vi "弹窗-手动静音.vi"(6 "引用-报警方式值改变？":refnum<vi>, 8 "引用-报警状态":refnum<vi>, 9 "引用-暂停发送":refnum<vi>, 10 "引用-报警方式":refnum<vi>, 11 "引用-实时数据列表":refnum<vi>) -> ()   [LabVIEW 2017]
panel:
  in  "列表框":i32(listbox)
  in  "事件-选中行":refnum<user-event>
  in  "选中行":i32[](array[numeric])
  out "项数":i32
  out "信号-刷新列表":bool=TRUE
  in  "上翻":bool
  in  "全部静音":bool
  in  "下翻":bool
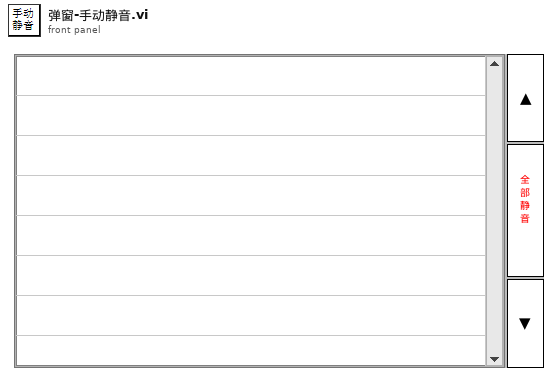
[diagram p1: front panel]
types:
  T1 = cluster{"报警方式":enum16{"常报警", "自动静音", "手动静音"}, "延迟计时":u16, "报警中？":bool}[]
  T2 = enum32{"Invalid", "Standard", "Closed", "Hidden", "Minimized", "Maximized"}
  T3 = cluster{"报警方式":enum16{"常报警", "自动静音", "手动静音"}, "延迟计时":u16, "报警中？":bool}
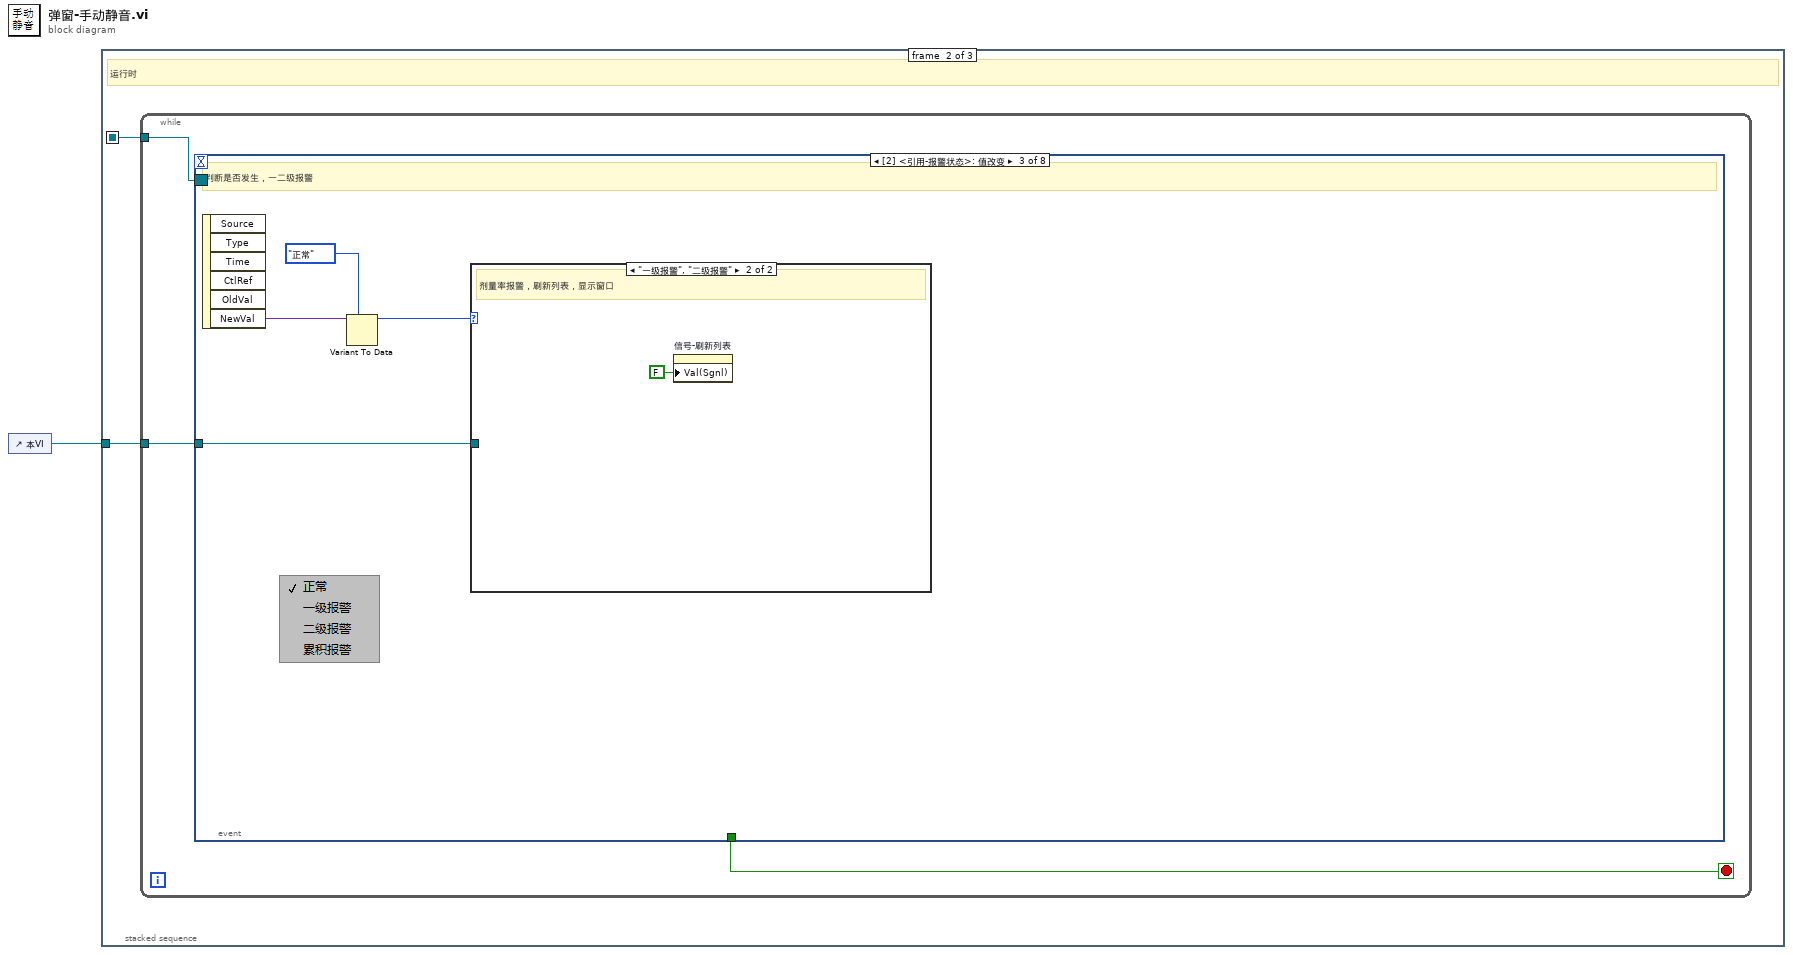
[diagram p0: block diagram]
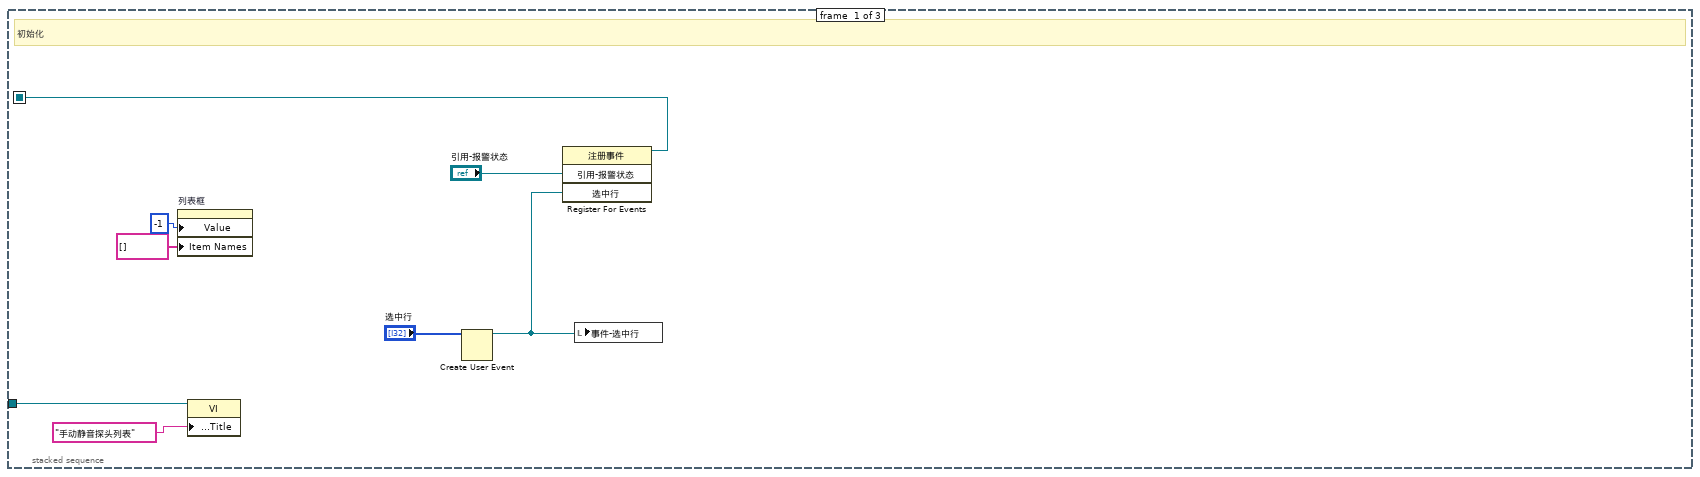
[diagram p2: hidden frame]
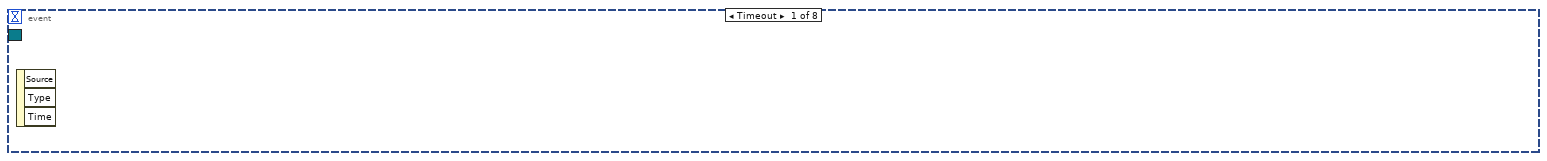
[diagram p3: hidden frame]
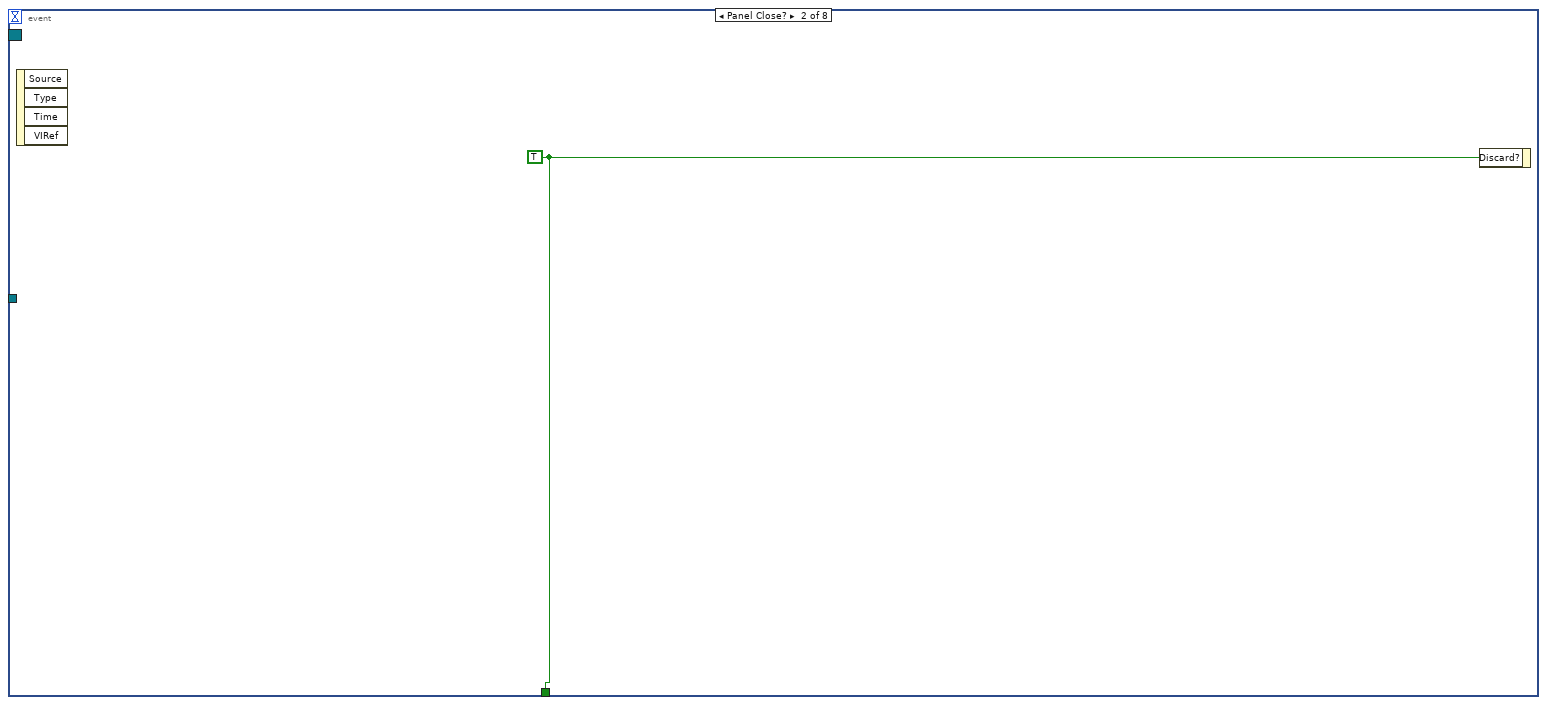
[diagram p4: hidden frame]
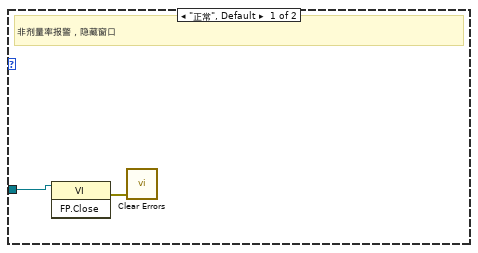
[diagram p5: hidden frame]
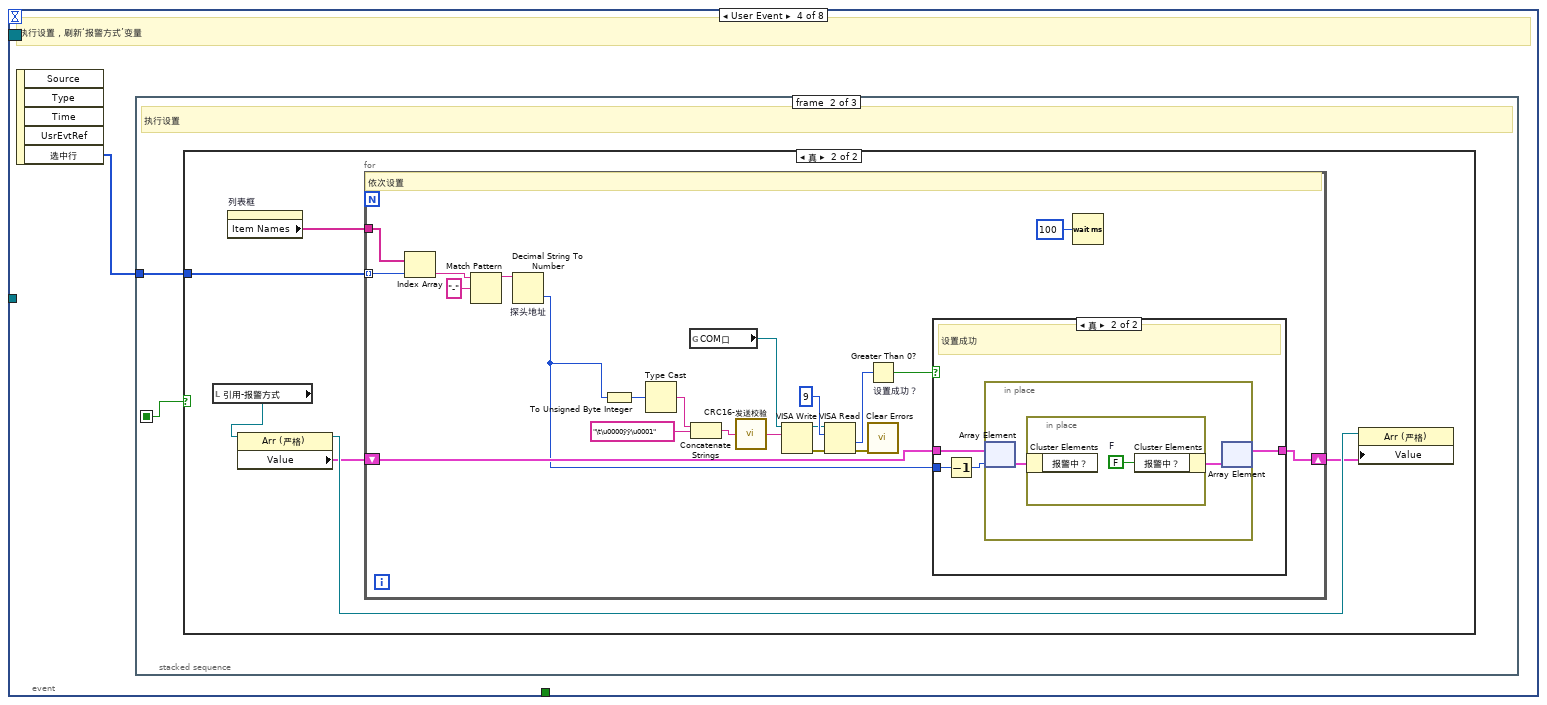
[diagram p6: hidden frame]
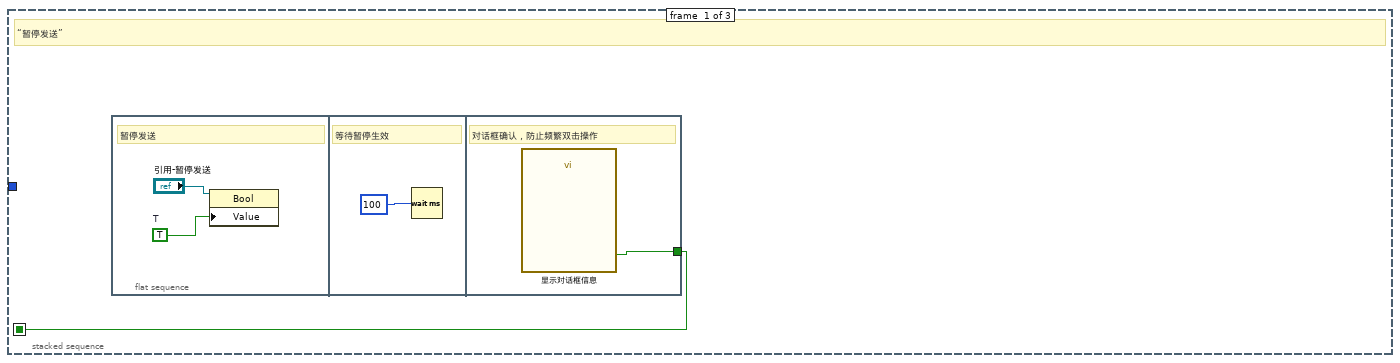
[diagram p7: hidden frame]
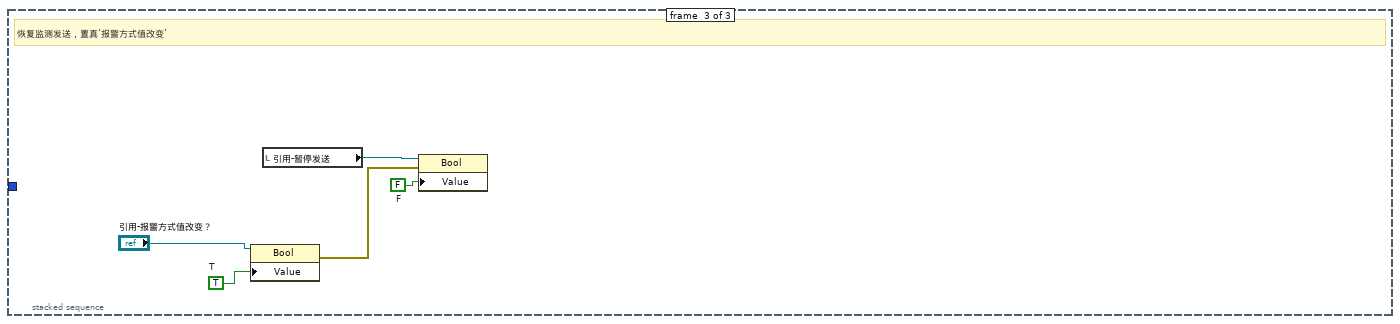
[diagram p10: hidden frame]
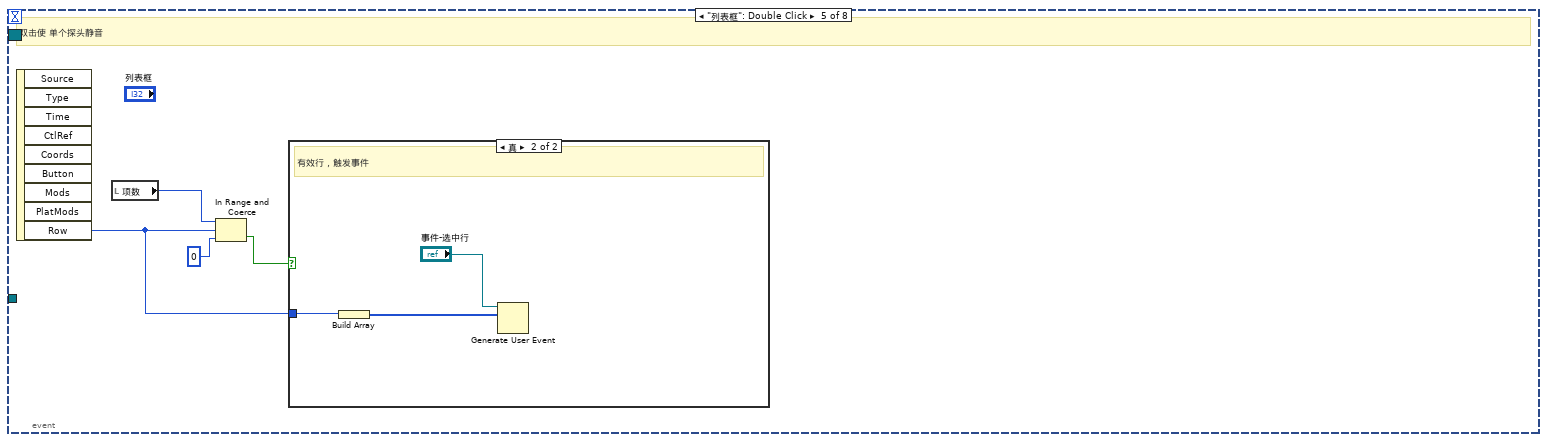
[diagram p11: hidden frame]
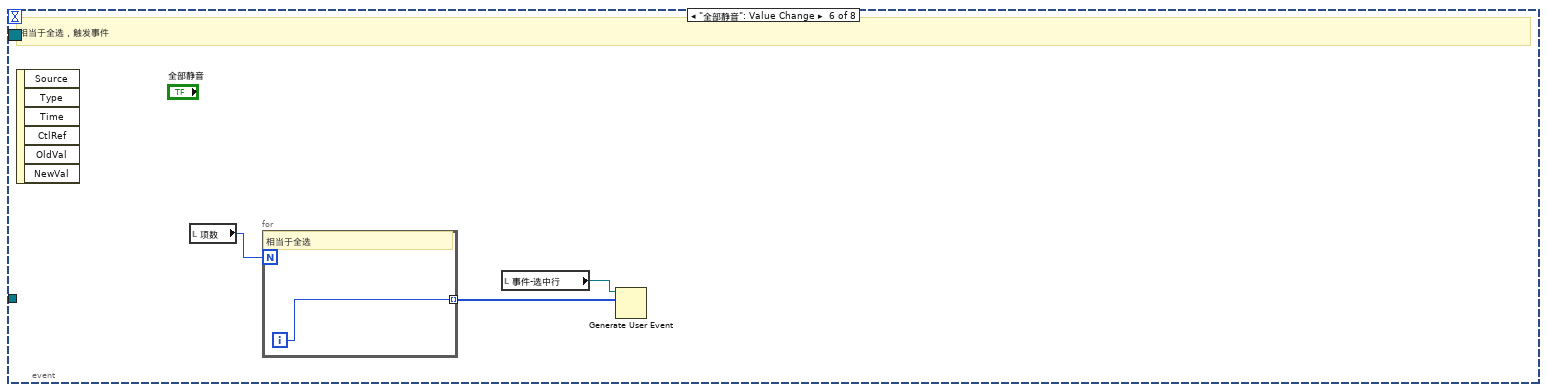
[diagram p13: hidden frame]
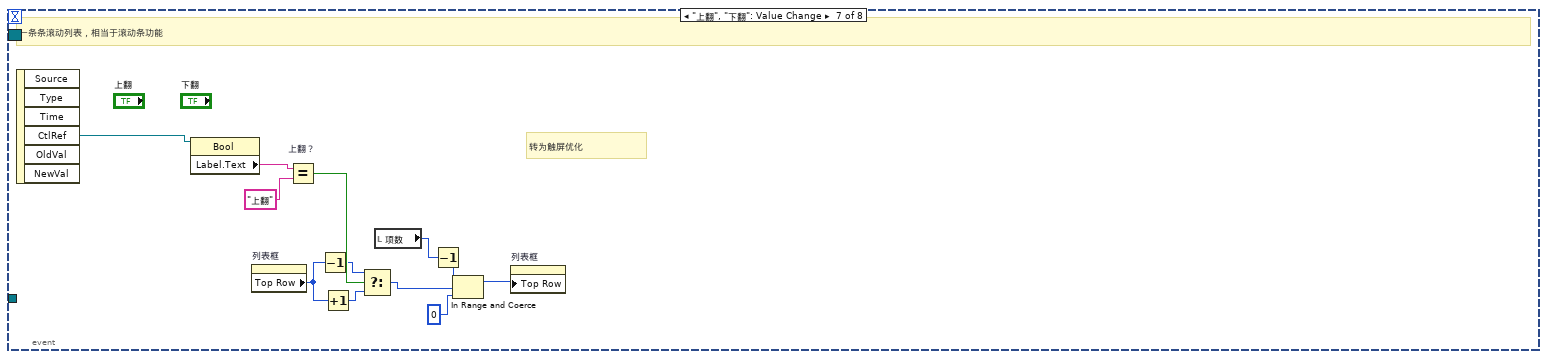
[diagram p14: hidden frame]
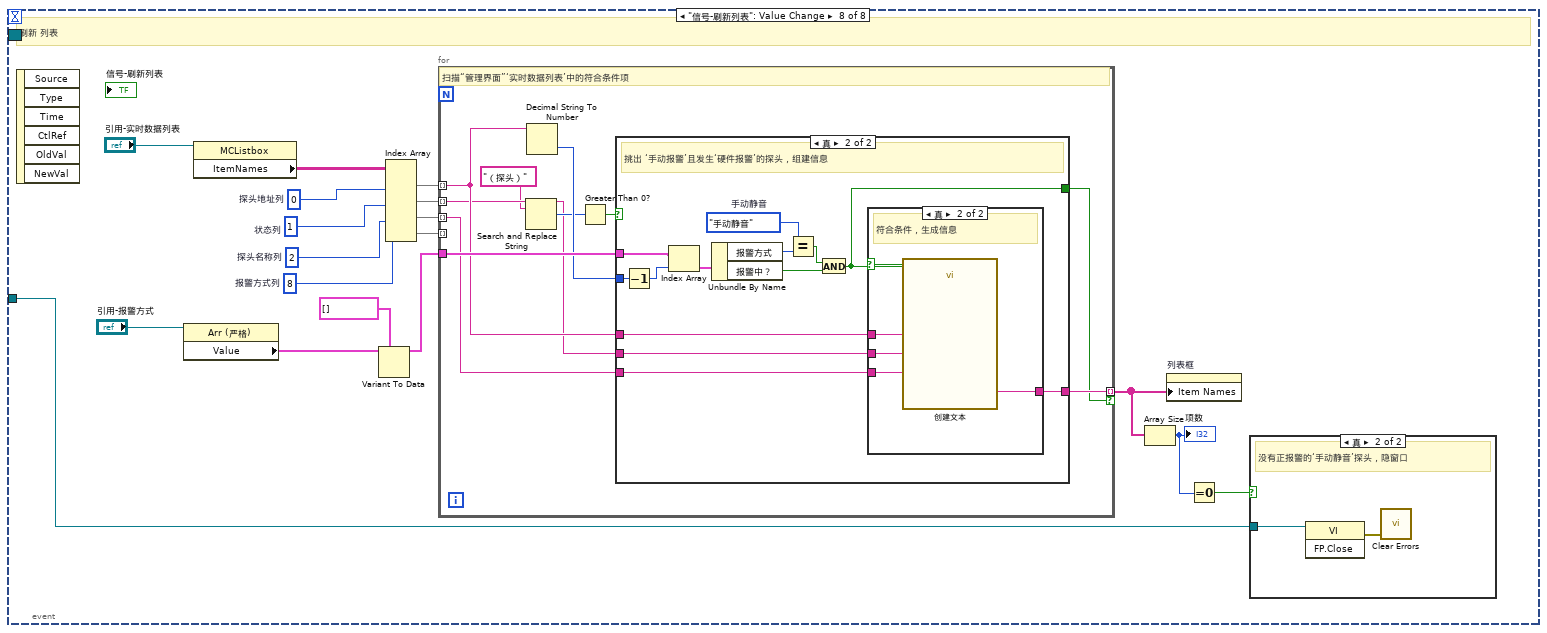
[diagram p15: hidden frame]
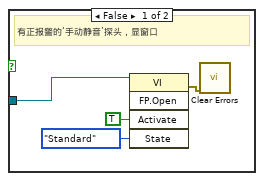
[diagram p16: hidden frame]
diagram:
  n1 = control-ref of="本VI"() -> (w1:refnum<vi>)
  n2 = stacked-sequence {
    seq-local: [w7 _ _] -> [_ w11 _]
    tunnel: w1 -> [w9 w10 _]
    frame #0 {
      # "初始化"
      n3 = property on="列表框" class="LstBox (严格)"("Value"=-1 ("列表框"), "Item Names"=string[] [] ("项名")) -> ()  [unwired: 2 in, 2 out]
      n4 = property class="VI"(reference=w9, "Front Panel.Title"="手动静音探头列表" ("前面板窗口:标题")) -> ()  [unwired: 1 in, 2 out]
      n5 = Create User Event(user event datatype="选中行") -> (user event=w2:refnum<user-event>)  [unwired: 1 in, 1 out]
      n6 = register-events("引用-报警状态", w2) -> (reference out=w7:refnum<event-registration>)  [unwired: 2 in, 1 out]
      n7 = local write "事件-选中行"(w2) -> ()
    }
    frame #1 {
      # "运行时"
      n8 = while {
        tunnel: w11 -> [w13]
        tunnel: w10 -> [w12]
        stop <- w14 stop-if-true
        n9 = event shown="[2] <引用-报警状态>: 值改变" {
          selector: w13 -> [_ _ _ _ _ _ _ _]
          dyn-events: _ -> [_ _ _ _ _ _ _ _]
          timeout: _ -> [_ _ _ _ _ _ _ _]
          tunnel: [_ w15 _ _ _ _ _ _] -> w14
          tunnel: w12 -> [_ _ w16 _ _ _ _ w94]
          event Timeout {
            n10 = event-data() -> ()  [unwired: 1 in, 3 out]
          }
          event Panel Close? {
            w15 = TRUE ("放弃？")
            n11 = event-data() -> ()  [unwired: 1 in, 4 out]
            n12 = event-data("Discard?"=w15) -> ()  [unwired: 1 in, 1 out]
          }
          event Value Change {
            # "判断是否发生，一二级报警"
            n13 = event-data() -> ("NewVal"=w17:variant)  [unwired: 1 in, 5 out]
            n14 = Variant To Data(type=enum16{"正常", "一级报警", "二级报警", "累积报警"}."正常" ("报警状态"), Variant=w17) -> (data=w18:enum16{"正常", "一级报警", "二级报警", "累积报警"})  [unwired: 1 in, 1 out]
            n15 = case shown="\"一级报警\", \"二级报警\"" w18 {
              tunnel: w16 -> [w20 _]
              frame "正常", Default {
                # "非剂量率报警，隐藏窗口"
                n16 = invoke class="VI" method="FP.Close"(reference=w20) -> (error out=w21:errorcluster)  [unwired: 2 in, 2 out]
                n17 = call <vilib>:"Clear Errors.vi"("error in (no error)"=w21) -> ()  [unwired: 5 in, 2 out]
              }
              frame "一级报警", "二级报警" {
                # "剂量率报警，刷新列表，显示窗口"
                n18 = property on="信号-刷新列表" class="Bool (严格)"("Val(Sgnl)"=FALSE ("值(信号)")) -> ()  [unwired: 2 in, 2 out]
              }
            }
          }
          event User Event {
            # "执行设置，刷新‘报警方式’变量"
            n19 = event-data() -> ("选中行"=w23:i32[])  [unwired: 1 in, 4 out]
            n20 = stacked-sequence {
              seq-local: [w24 _ _] -> [_ w29 _]
              tunnel: w23 -> [_ w30 _]
              frame #0 {
                # "“暂停发送”"
                n21 = flat-sequence {
                  tunnel: [w28] -> w24
                  frame #0 {
                    w25 = TRUE  # T
                    # "暂停发送"
                    n22 = property class="Bool"(reference="引用-暂停发送", "Value"=w25) -> ()  [unwired: 1 in, 2 out]
                  }
                  frame #1 {
                    # "等待暂停生效"
                    n23 = Wait (ms)(milliseconds to wait=u32 100 ("等待时间（毫秒）")) -> ()  [unwired: 1 out]
                  }
                  frame #2 {
                    # "对话框确认，防止频繁双击操作"
                    n24 = call "显示对话框信息"() -> ("确定"=w28:bool)  [unwired: 10 in, 1 out]
                  }
                }
              }
              frame #1 {
                # "执行设置"
                n25 = case shown="真" w29 {
                  tunnel: w30 -> [_ w34]
                  frame False {
                  }
                  frame True {
                    n26 = local read "引用-报警方式"() -> (w36:refnum<vi>)
                    n27 = property on="列表框" class="LstBox (严格)"() -> ("Item Names"=w31:string[])  [unwired: 2 in, 2 out]
                    n28 = property class="Arr (严格)"(reference=w36) -> (reference out=w35:refnum<vi>, "Value"=w33:T1)  [unwired: 1 in, 1 out]
                    n29 = for {
                      tunnel: w34 -> [w40] mode=indexing
                      shift-right: [w39] -> w32
                      shift-left: w33 -> [w41]
                      tunnel: w31 -> [w57]
                      # "依次设置"
                      n30 = Index Array(array=w57, index=w40) -> (element=w56:string)
                      n31 = Match Pattern(string=w56, regular expression="-" ("正则表达式")) -> (before substring=w54:string)  [unwired: 1 in, 3 out]
                      n32 = Decimal String To Number "探头地址"(string=w54) -> (number=w37:i32)  [unwired: 2 in, 1 out]
                      n33 = To Unsigned Byte Integer(number=w37) -> (unsigned 8bit integer=w52:u8)
                      n34 = Type Cast(x=w52) -> (*(type *) &x=w53:string)  [unwired: 1 in]
                      n35 = global read "全局变量-35点监测.vi" "COM口"() -> (w38:refnum<visa-resource-name>)
                      n36 = Concatenate Strings(w53, "\t\u0000ÿÿ\u0001") -> (w44:string)
                      n37 = call "CRC16-发送校验.vi"("净数据"=w44) -> ("完整输出"=w45:string)
                      n38 = VISA Write(VISA resource name=w38, write buffer=w45) -> (VISA resource name out=w47:refnum<visa-resource-name>, error out=w46:errorcluster)  [unwired: 1 in, 1 out]
                      n39 = VISA Read(VISA resource name=w47, byte count=u32 9 ("字节总数"), error in (no error)=w46) -> (return count=w49:u32, error out=w50:errorcluster)  [unwired: 2 out]
                      n40 = Greater Than 0? "设置成功？"(x=w49) -> (x > 0?=w43:bool)
                      n41 = call <vilib>:"Clear Errors.vi"("error in (no error)"=w50) -> ()  [unwired: 5 in, 2 out]
                      n42 = case shown="真" w43 {
                        tunnel: w41 -> [w58 w62]
                        tunnel: w37 -> [_ w60]
                        tunnel: [w58 w59] -> w39
                        frame False {
                          # "不改变值"
                        }
                        frame True {
                          # "设置成功"
                          n43 = Decrement(x=w60) -> (x-1=w61:i32)
                          n44 = in-place {
                            n45 = in-place-array #1(w62, w61) -> (w64:T3)
                            n46 = in-place {
                              w65 = FALSE  # F
                              n47 = in-place-cluster #2(w64) -> ()  [unwired: 1 out]
                              n48 = in-place-cluster #2("报警中？"=w65) -> (w63:T3)
                            }
                            n49 = in-place-array #1(w63) -> (w59:T1)  [unwired: 1 out]
                          }
                        }
                      }
                      n50 = Wait (ms)(milliseconds to wait=u32 100 ("等待时间（毫秒）")) -> ()  [unwired: 1 out]
                    }
                    n51 = property class="Arr (严格)"(reference=w35, "Value"=w32) -> ()  [unwired: 1 in, 2 out]
                  }
                }
              }
              frame #2 {
                w67 = TRUE  # T
                w70 = FALSE  # F
                # "恢复监测发送，置真‘报警方式值改变’"
                n52 = property class="Bool"(reference="引用-报警方式值改变？", "Value"=w67) -> (error out=w66:errorcluster)  [unwired: 1 in, 1 out]
                n53 = local read "引用-暂停发送"() -> (w69:refnum<vi>)
                n54 = property class="Bool"(reference=w69, error in=w66, "Value"=w70) -> ()  [unwired: 2 out]
              }
            }
          }
          event "列表框": Double Click {
            # "双击使 单个探头静音"
            n55 = event-data() -> ("Row"=w71:i32)  [unwired: 1 in, 8 out]
            n56 = local read "项数"() -> (w73:i32)
            n57 = In Range and Coerce(upper limit=w73, x=w71, lower limit=0 ("下限")) -> (In Range?=w72:bool)  [unwired: 1 out]
            n58 = case shown="真" w72 {
              tunnel: w71 -> [_ w77]
              frame False {
                # "无效行"
              }
              frame True {
                # "有效行，触发事件"
                n59 = Build Array(w77) -> (w75:i32[])
                n60 = Generate User Event(user event="事件-选中行", event data cluster=w75) -> ()  [unwired: 2 in, 2 out]
              }
            }
          }
          event "全部静音": Value Change {
            # "相当于全选，触发事件"
            n61 = event-data() -> ()  [unwired: 1 in, 6 out]
            n62 = local read "项数"() -> (w80:i32)
            n63 = for {
              N: w80 -> [_]
              tunnel: [w81] -> w79 mode=indexing
              i -> [w81]
              # "相当于全选"
            }
            n64 = local read "事件-选中行"() -> (w78:refnum<user-event>)
            n65 = Generate User Event(user event=w78, event data cluster=w79) -> ()  [unwired: 2 in, 2 out]
          }
          event "上翻", "下翻": Value Change {
            # "转为触屏优化"
            # "一条条滚动列表，相当于滚动条功能"
            n66 = event-data() -> ("CtlRef"=w93:refnum<vi>)  [unwired: 1 in, 5 out]
            n67 = property class="Bool"(reference=w93) -> ("Label.Text"=w92:string)  [unwired: 1 in, 2 out]
            n68 = property on="列表框" class="LstBox (严格)"() -> ("Top Row"=w86:i32)  [unwired: 2 in, 2 out]
            n69 = Equal? "上翻？"(x=w92, y="上翻") -> (x = y?=w88:bool)
            n70 = Decrement(x=w86) -> (x-1=w87:i32)
            n71 = Increment(x=w86) -> (x+1=w85:i32)
            n72 = Select(t=w87, s=w88, f=w85) -> (s? t:f=w84:i32)
            n73 = local read "项数"() -> (w90:i32)
            n74 = Decrement(x=w90) -> (x-1=w82:i32)
            n75 = In Range and Coerce(upper limit=w82, x=w84, lower limit=0 ("下限")) -> (coerced(x)=w83:i32)  [unwired: 1 out]
            n76 = property on="列表框" class="LstBox (严格)"("Top Row"=w83) -> ()  [unwired: 2 in, 2 out]
          }
          event "信号-刷新列表": Value Change {
            w103 = 8  # 报警方式列
            w102 = 2  # 探头名称列
            w101 = 1  # 状态列
            w100 = 0  # 探头地址列
            # "刷新 列表"
            n77 = event-data() -> ()  [unwired: 1 in, 6 out]
            n78 = property class="Arr (严格)"(reference="引用-报警方式") -> ("Value"=w110:T1)  [unwired: 1 in, 2 out]
            n79 = property class="MCListbox"(reference="引用-实时数据列表") -> ("ItemNames"=w99:string[][])  [unwired: 1 in, 2 out]
            n80 = Variant To Data(type=T1 [] ("报警方式"), Variant=w110) -> (data=w111:T1)  [unwired: 1 in, 1 out]
            n81 = Index Array(array=w99, index (col) #1=w100, index (col) #2=w101, index (col) #3=w102, index (col) #4=w103) -> (element #1=w107:string[], element #2=w106:string[], element #3=w105:string[], element #4=w104:string[])  [unwired: 4 in]
            n82 = for {
              tunnel: w104 -> [_] mode=indexing
              tunnel: w105 -> [w125] mode=indexing
              tunnel: w106 -> [w122] mode=indexing
              tunnel: w107 -> [w126] mode=indexing
              tunnel: w111 -> [w128]
              tunnel: [w124] -> w97 mode=indexing if=w123
              # "扫描“管理界面”‘实时数据列表’中的符合条件项"
              n83 = Search and Replace String(input string=w122, search string="（探头）") -> (result string=w118:string, number of replacements=w120:i32)  [unwired: 6 in, 2 out]
              n84 = Decimal String To Number(string=w126) -> (number=w127:i32)  [unwired: 2 in, 1 out]
              n85 = Greater Than 0?(x=w120) -> (x > 0?=w119:bool)
              n86 = case shown="真" w119 {
                tunnel: w128 -> [_ w140]
                tunnel: w127 -> [_ w134]
                tunnel: w126 -> [_ w133]
                tunnel: w125 -> [_ w132]
                tunnel: [_ w131] -> w124
                tunnel: [_ w130] -> w123
                tunnel: w118 -> [_ w129]
                frame False {
                }
                frame True {
                  w136 = enum16{"常报警", "自动静音", "手动静音"}."手动静音"  # 手动静音
                  # "挑出 ‘手动报警’且发生‘硬件报警’的探头，组建信息"
                  n87 = Decrement(x=w134) -> (x-1=w141:i32)
                  n88 = Index Array(array=w140, index=w141) -> (element=w139:T3)
                  n89 = Unbundle By Name(w139) -> ("报警方式"=w137:enum16{"常报警", "自动静音", "手动静音"}, "报警中？"=w138:bool)
                  n90 = Equal?(x=w136, y=w137) -> (x = y?=w135:bool)
                  n91 = And(x=w135, y=w138) -> (x .and. y?=w130:bool)
                  n92 = case shown="真" w130 {
                    tunnel: w133 -> [_ w145]
                    tunnel: w129 -> [_ w144]
                    tunnel: w132 -> [_ w143]
                    tunnel: [_ w142] -> w131
                    frame False {
                      # "不符合条件"
                    }
                    frame True {
                      # "符合条件，生成信息"
                      n93 = call "创建文本"("探头地址"=w145, "报警等级"=w144, "探头名称"=w143) -> ("Result"=w142:string)  [unwired: 11 in, 1 out]
                    }
                  }
                }
              }
            }
            n94 = Array Size(array=w97) -> (size(s)=w96:i32)
            "项数" <- w96
            n95 = property on="列表框" class="LstBox (严格)"("Item Names"=w97) -> ()  [unwired: 2 in, 2 out]
            n96 = Equal To 0?(x=w96) -> (x = 0?=w95:bool)
            n97 = case shown="真" w95 {
              tunnel: w94 -> [w112 w117]
              frame False {
                # "有正报警的‘手动静音’探头，显窗口"
                n98 = invoke class="VI" method="FP.Open"(reference=w112, "Activate"=TRUE ("激活？"), "State"=T2."Standard" ("状态")) -> (error out=w113:errorcluster)  [unwired: 2 in, 4 out]
                n99 = call <vilib>:"Clear Errors.vi"("error in (no error)"=w113) -> ()  [unwired: 5 in, 2 out]
              }
              frame True {
                # "没有正报警的‘手动静音’探头，隐窗口"
                n100 = invoke class="VI" method="FP.Close"(reference=w117) -> (error out=w116:errorcluster)  [unwired: 2 in, 2 out]
                n101 = call <vilib>:"Clear Errors.vi"("error in (no error)"=w116) -> ()  [unwired: 5 in, 2 out]
              }
            }
          }
        }
      }
    }
    frame #2 {
      # "结束"
    }
  }
